vi "EventsRobotsStuck.vi"(6 "IA State Input":T5, 9 "Time":enum16{"Azul", "Amarelo"}(ring), 10 "Single frame":T1 {"robots_blue"."height" format="%+4.3f"; "robots_blue"."pixel_y" format="%+4.3f"; "robots_blue"."pixel_x" format="%+4.3f"; "robots_blue"."orientation" format="%+4.3f"; "robots_blue"."y" format="%+4.3f"; "robots_blue"."confidence" format="%4.3f"; "robots_blue"."x" format="%+4.3f"; "robots_yellow"."height" format="%+4.3f"; "robots_yellow"."pixel_y" format="%+4.3f"; "robots_yellow"."pixel_x" format="%+4.3f"; "robots_yellow"."orientation" format="%+4.3f"; "robots_yellow"."y" format="%+4.3f"; "robots_yellow"."confidence" format="%4.3f"; "robots_yellow"."x" format="%+4.3f"}, 11 "fps":dbl) -> ()   [LabVIEW 2017]
uses:
  Core/AI Input.ctl
  Core/AI Robot.ctl
  Intel/Functions Enum.ctl
  Intel/AttackerStates.ctl
  Path Planning/RRT/PathDests.ctl
  Path Planning/RRT/PathDest.ctl
  Core/AI Ball.ctl
  Core/Field Size.ctl
  Core/AI Judge.ctl
  Intel/Command Enum.ctl
  Events.ctl
  SSL Detection Frame.ctl
  SSL Detection Robot.ctl
  <vilib>/Analysis/Matrix/Datatypes/RealMatrix.ctl
  SSL Detection Ball.ctl
  <vilib>/Analysis/Matrix/NI_Matrix.lvlib
panel:
  out "Robots Stucked":cluster{"ID":i32, "Relative error":dbl}[](array[cluster])
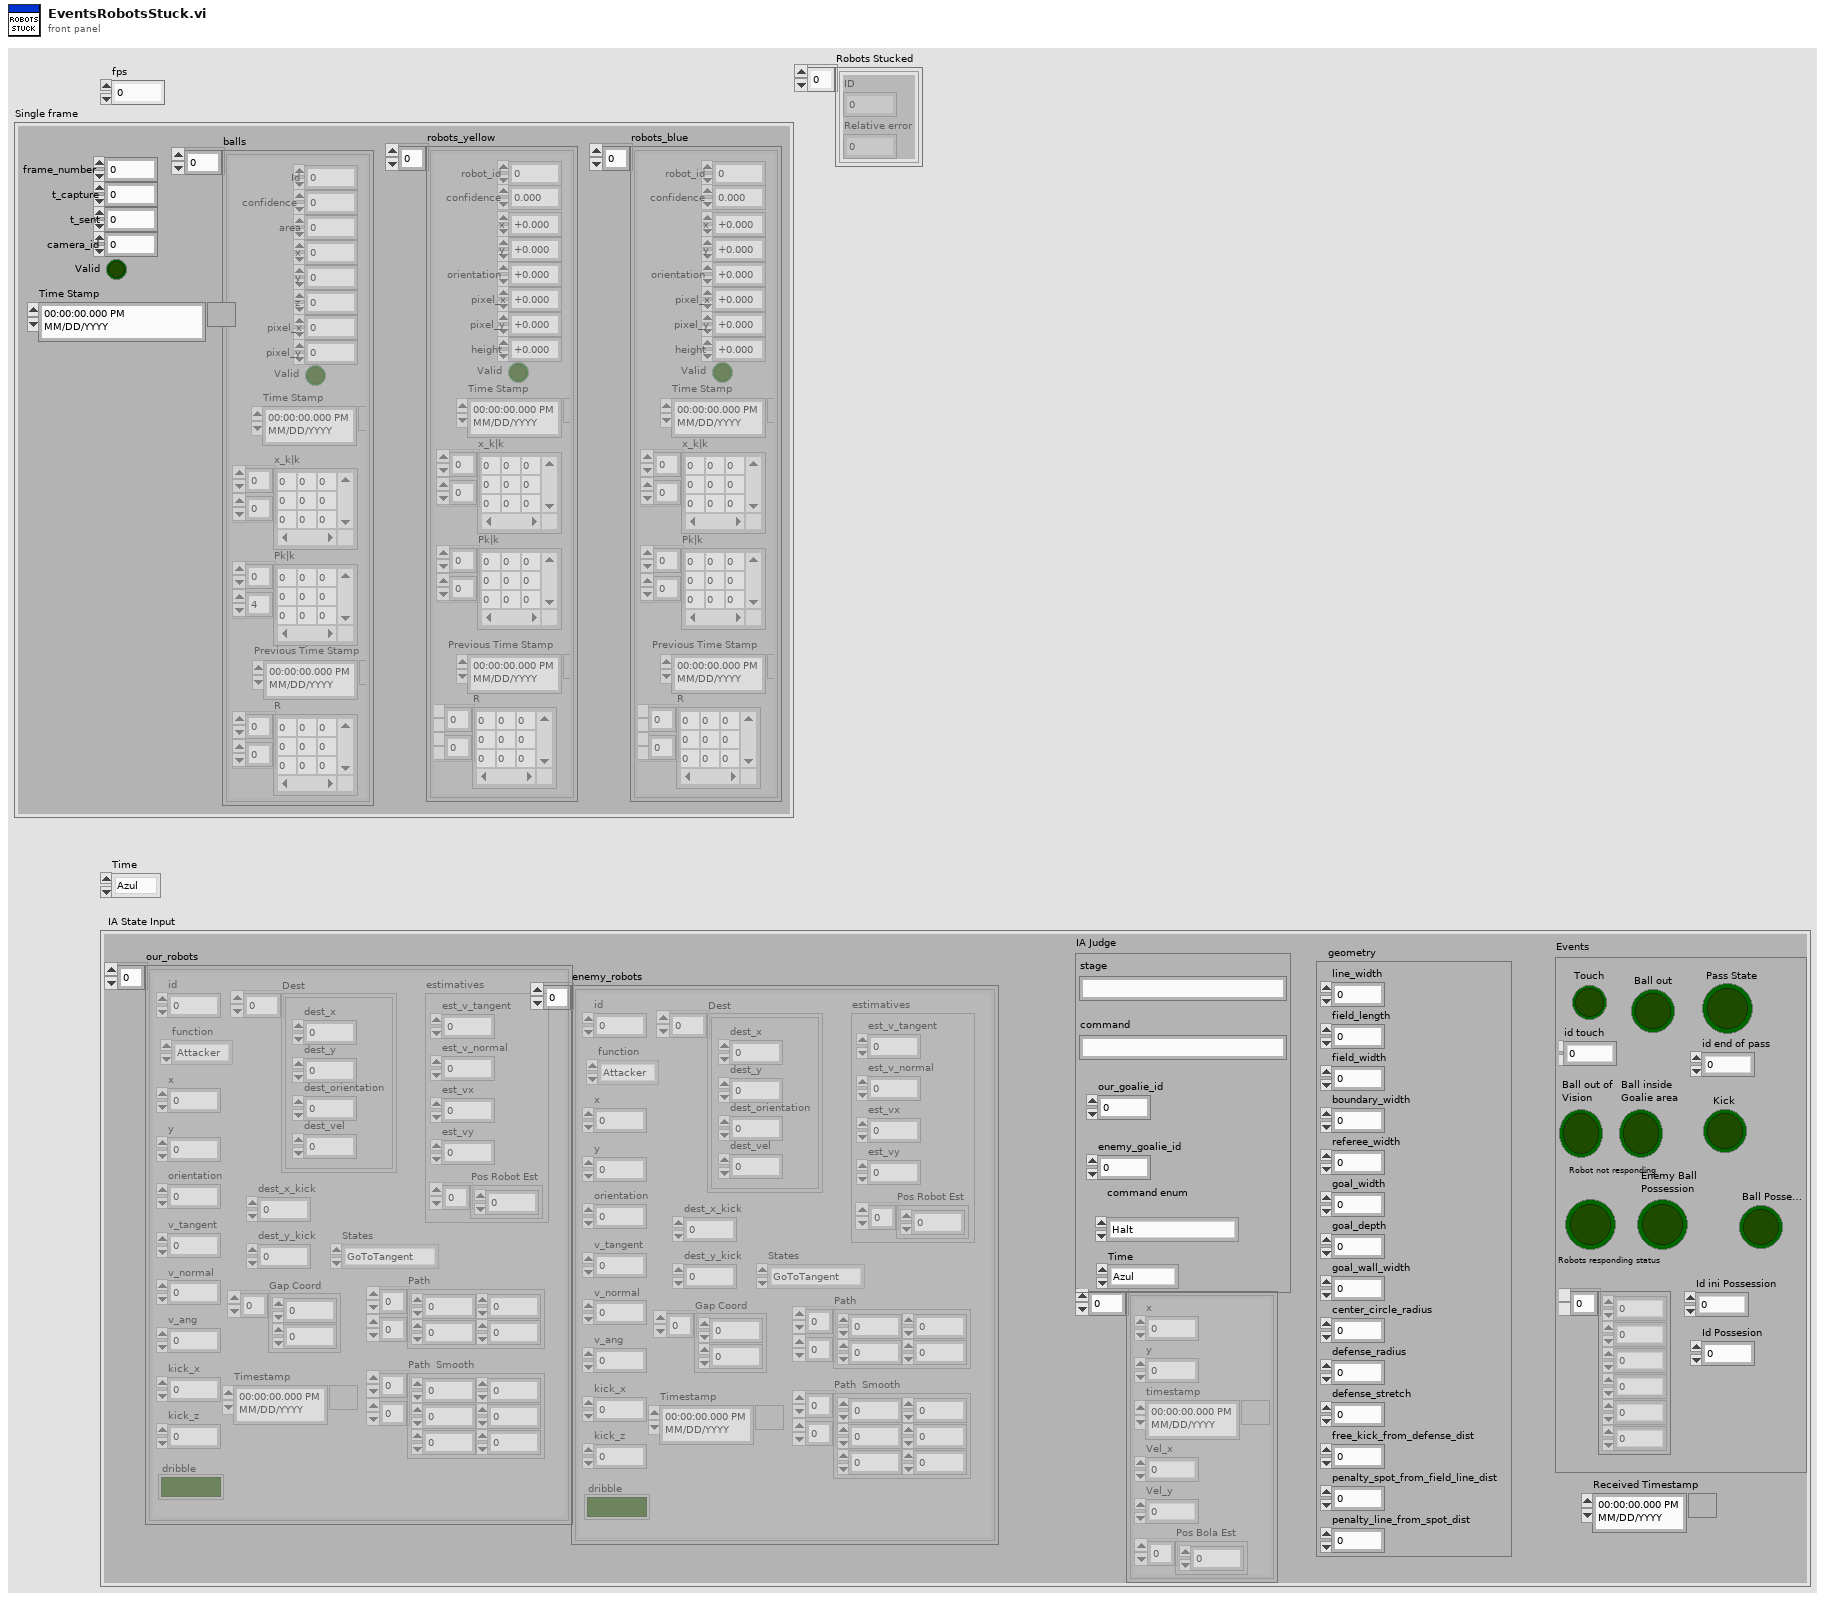
[diagram p1: front panel]
types:
  T1 = typedef "SSL Detection Frame.ctl" = cluster{"frame_number":u32, "t_capture":dbl, "t_sent":dbl, "camera_id":u32, "robots_yellow":T2[], "robots_blue":T2[], "balls":T4[], "Valid":bool, "Time Stamp":timestamp}
  T2 = typedef "SSL Detection Robot.ctl" = cluster{"x":sgl, "robot_id":u32, "confidence":sgl, "y":sgl, "orientation":sgl, "pixel_x":sgl, "pixel_y":sgl, "height":sgl, "Valid":bool, "Time Stamp":timestamp, "x_k|k":T3, "Pk|k":T3, "Previous Time Stamp":timestamp, "R":T3}
  T3 = typedef "NI_Matrix.lvlib/RealMatrix.ctl" = dbl[][]
  T4 = typedef "SSL Detection Ball.ctl" = cluster{"x":sgl, "area":u32, "confidence":sgl, "y":sgl, "z":sgl, "pixel_x":sgl, "pixel_y":sgl, "Valid":bool, "Time Stamp":timestamp, "x_k|k":T3, "Pk|k":T3, "Id":u32, "Previous Time Stamp":timestamp, "R":T3}
  T5 = typedef "AI Input.ctl" = cluster{"our_robots":T6[], "enemy_robots":T6[], "balls":T11[], "geometry":T12, "IA Judge":T13, "Received Timestamp":timestamp, "Events":T15}
  T6 = typedef "AI Robot.ctl" = cluster{"id":u32, "function":T7, "x":dbl, "y":dbl, "orientation":dbl, "v_tangent":dbl, "v_normal":dbl, "v_ang":dbl, "kick_x":dbl, "kick_z":dbl, "dribble":bool, "Timestamp":timestamp, "estimatives":cluster{"est_v_tangent":dbl, "est_v_normal":dbl, "est_vx":dbl, "est_vy":dbl, "Pos Robot Est":dbl[]}, "dest_x_kick":dbl, "dest_y_kick":dbl, "Gap Coord":dbl[], "States":T8, "Path ":dbl[][], "Path  Smooth":dbl[][], "Dest":T9}
  T7 = typedef "Functions Enum.ctl" = enum16{"Attacker", "Goalie", "Defender", "Striker", "Goto 0", "Dummy", "Kicker", "ZigZag"}
  T8 = typedef "AttackerStates.ctl" = enum16{"Pass", "GoToTangent", "BallGetting", "GoToKick", ""}
  T9 = typedef "PathDests.ctl" = T10[]
  T10 = typedef "PathDest.ctl" = cluster{"dest_x":dbl, "dest_y":dbl, "dest_orientation":dbl, "dest_vel":dbl}
  T11 = typedef "AI Ball.ctl" = cluster{"x":dbl, "y":dbl, "timestamp":timestamp, "Vel_x":dbl, "Vel_y":dbl, "Pos Bola Est":dbl[]}
  T12 = typedef "Field Size.ctl" = cluster{"line_width":u32, "field_length":u32, "field_width":u32, "boundary_width":u32, "referee_width":u32, "goal_width":u32, "goal_depth":u32, "goal_wall_width":u32, "center_circle_radius":u32, "defense_radius":u32, "defense_stretch":u32, "free_kick_from_defense_dist":u32, "penalty_spot_from_field_line_dist":u32, "penalty_line_from_spot_dist":u32}
  T13 = typedef "AI Judge.ctl" = cluster{"stage":string, "command":string, "our_goalie_id":dbl, "enemy_goalie_id":dbl, "command enum":T14, "Time":enum16{"Azul", "Amarelo"}}
  T14 = typedef "Command Enum.ctl" = enum16{"Halt", "Stop", "Force Start", "PKA Normal Start", "Prepare Kickoff Ally", "PKE Normal Start", "Prepare Kickoff Enemy", "Prepare Penalty Ally", "PPA Normal Start", "Prepare Penalty Enemy", "PPE Normal Start", "Direct Free Enemy", "Direct Free Ally", "Indirect Free Enemy", "Indirect Free Ally", "Timeout Enemy", "Timeout Ally", "Goal Enemy", "Goal Ally", "Ball Placement Enemy", "Ball Placement Ally", "Normal Half Time", "Extra Time Break", "Extra Half Time", "None", "Post Game"}
  T15 = typedef "Events.ctl" = cluster{"Touch":bool, "Ball out":bool, "id touch":dbl, "Ball out of \nVision":bool, "Ball inside \nGoalie area":bool, "Robot not responding":bool, "Robots responding status":dbl[], "Enemy Ball \nPossession":bool, "Pass State":bool, "id end of pass":dbl, "Kick":bool, "Id ini Possession":dbl, "Ball Possesion":bool, "Id Possesion":dbl}
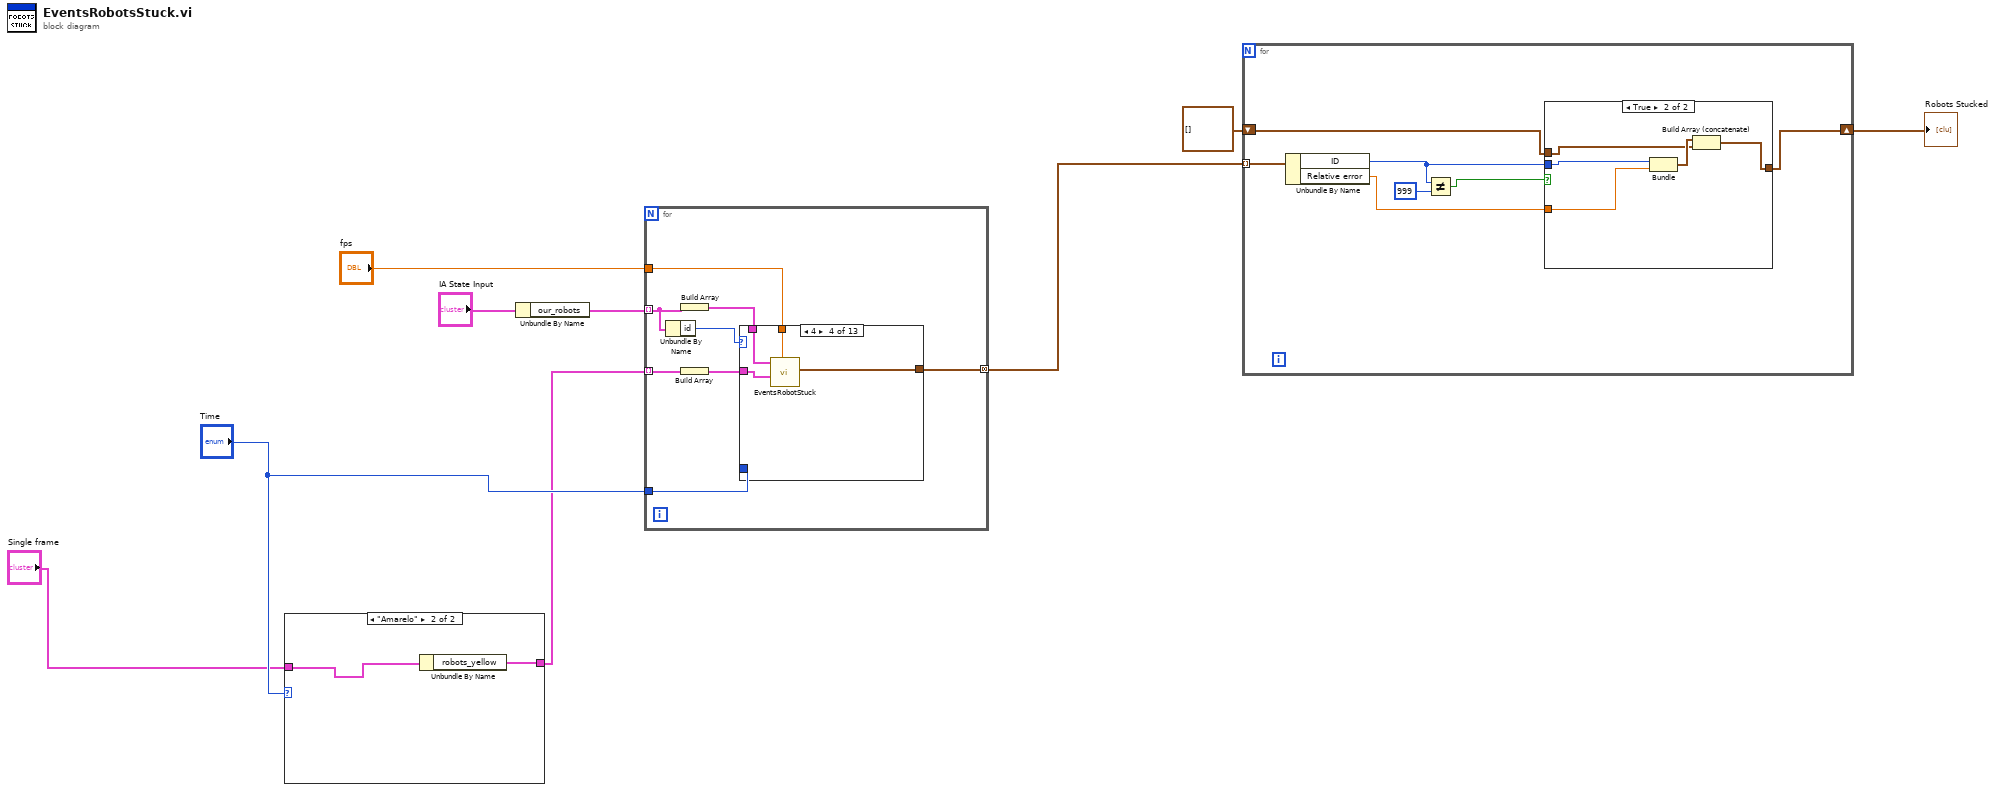
[diagram p0: block diagram]
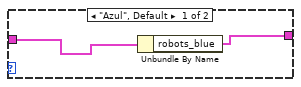
[diagram p3: hidden frame]
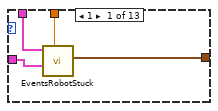
[diagram p4: hidden frame]
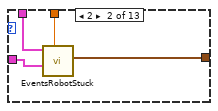
[diagram p5: hidden frame]
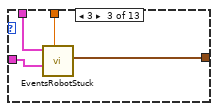
[diagram p6: hidden frame]
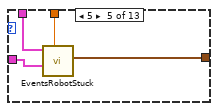
[diagram p7: hidden frame]
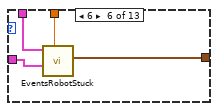
[diagram p8: hidden frame]
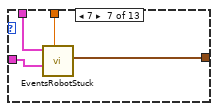
[diagram p9: hidden frame]
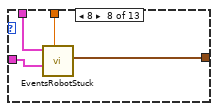
[diagram p10: hidden frame]
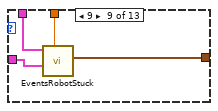
[diagram p11: hidden frame]
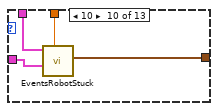
[diagram p12: hidden frame]
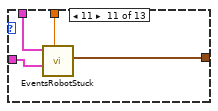
[diagram p13: hidden frame]
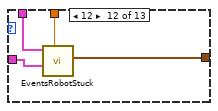
[diagram p14: hidden frame]
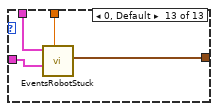
[diagram p15: hidden frame]
diagram:
  n1 = case shown="\"Amarelo\"" "Time" {
    tunnel: "Single frame" -> [w10 w12]
    tunnel: [w11 w13] -> w5
    frame "Azul", Default {
      n2 = Unbundle By Name(w10) -> ("robots_blue"=w11:T2[])
    }
    frame "Amarelo" {
      n3 = Unbundle By Name(w12) -> ("robots_yellow"=w13:T2[])
    }
  }
  n4 = Unbundle By Name("IA State Input") -> ("our_robots"=w7:T6[])
  n5 = for {
    tunnel: "fps" -> [w21]
    tunnel: "Time" -> [w20]
    tunnel: w7 -> [w17] mode=indexing
    tunnel: w5 -> [w15] mode=indexing
    tunnel: [w14] -> w3 mode=concatenating
    n6 = Unbundle By Name(w17) -> ("id"=w16:u32)
    n7 = Build Array(w17) -> (w18:T6[])
    n8 = Build Array(w15) -> (w19:T2[])
    n9 = case shown="4" w16 {
      tunnel: w21 -> [w25 w29 w33 w37 w41 w45 w49 w53 w57 w61 w65 w69 w73]
      tunnel: w20 -> [_ _ _ _ _ _ _ _ _ _ _ _ _]
      tunnel: w19 -> [w23 w27 w31 w35 w39 w43 w47 w51 w55 w59 w63 w67 w71]
      tunnel: w18 -> [w24 w28 w32 w36 w40 w44 w48 w52 w56 w60 w64 w68 w72]
      tunnel: [w22 w26 w30 w34 w38 w42 w46 w50 w54 w58 w62 w66 w70] -> w14
      frame 1 {
        n10 = call "EventsRobotStuck.vi"("our_robots"=w24, "Our_Robots frame"=w23, "FPS"=w25) -> ("Array"=w22:cluster{"ID":i32, "Relative error":dbl}[])  [unwired: 7 in]
      }
      frame 2 {
        n11 = call "EventsRobotStuck.vi"("our_robots"=w28, "Our_Robots frame"=w27, "FPS"=w29) -> ("Array"=w26:cluster{"ID":i32, "Relative error":dbl}[])  [unwired: 7 in]
      }
      frame 3 {
        n12 = call "EventsRobotStuck.vi"("our_robots"=w32, "Our_Robots frame"=w31, "FPS"=w33) -> ("Array"=w30:cluster{"ID":i32, "Relative error":dbl}[])  [unwired: 7 in]
      }
      frame 4 {
        n13 = call "EventsRobotStuck.vi"("our_robots"=w36, "Our_Robots frame"=w35, "FPS"=w37) -> ("Array"=w34:cluster{"ID":i32, "Relative error":dbl}[])  [unwired: 7 in]
      }
      frame 5 {
        n14 = call "EventsRobotStuck.vi"("our_robots"=w40, "Our_Robots frame"=w39, "FPS"=w41) -> ("Array"=w38:cluster{"ID":i32, "Relative error":dbl}[])  [unwired: 7 in]
      }
      frame 6 {
        n15 = call "EventsRobotStuck.vi"("our_robots"=w44, "Our_Robots frame"=w43, "FPS"=w45) -> ("Array"=w42:cluster{"ID":i32, "Relative error":dbl}[])  [unwired: 7 in]
      }
      frame 7 {
        n16 = call "EventsRobotStuck.vi"("our_robots"=w48, "Our_Robots frame"=w47, "FPS"=w49) -> ("Array"=w46:cluster{"ID":i32, "Relative error":dbl}[])  [unwired: 7 in]
      }
      frame 8 {
        n17 = call "EventsRobotStuck.vi"("our_robots"=w52, "Our_Robots frame"=w51, "FPS"=w53) -> ("Array"=w50:cluster{"ID":i32, "Relative error":dbl}[])  [unwired: 7 in]
      }
      frame 9 {
        n18 = call "EventsRobotStuck.vi"("our_robots"=w56, "Our_Robots frame"=w55, "FPS"=w57) -> ("Array"=w54:cluster{"ID":i32, "Relative error":dbl}[])  [unwired: 7 in]
      }
      frame 10 {
        n19 = call "EventsRobotStuck.vi"("our_robots"=w60, "Our_Robots frame"=w59, "FPS"=w61) -> ("Array"=w58:cluster{"ID":i32, "Relative error":dbl}[])  [unwired: 7 in]
      }
      frame 11 {
        n20 = call "EventsRobotStuck.vi"("our_robots"=w64, "Our_Robots frame"=w63, "FPS"=w65) -> ("Array"=w62:cluster{"ID":i32, "Relative error":dbl}[])  [unwired: 7 in]
      }
      frame 12 {
        n21 = call "EventsRobotStuck.vi"("our_robots"=w68, "Our_Robots frame"=w67, "FPS"=w69) -> ("Array"=w66:cluster{"ID":i32, "Relative error":dbl}[])  [unwired: 7 in]
      }
      frame 0, Default {
        n22 = call "EventsRobotStuck.vi"("our_robots"=w72, "Our_Robots frame"=w71, "FPS"=w73) -> ("Array"=w70:cluster{"ID":i32, "Relative error":dbl}[])  [unwired: 7 in]
      }
    }
  }
  n23 = for {
    tunnel: w3 -> [w80] mode=indexing
    shift-right: [w76] -> w1
    shift-left: cluster{"ID":i32, "Relative error":dbl}[] [] -> [w75]
    n24 = Unbundle By Name(w80) -> ("ID"=w77:i32, "Relative error"=w74:dbl)
    n25 = Not Equal?(x=w77, y=u32 999) -> (x != y?=w78:bool)
    n26 = case shown="True" w78 {
      tunnel: [w81 w84] -> w76
      tunnel: w77 -> [_ w86]
      tunnel: w75 -> [w81 w82]
      tunnel: w74 -> [_ w85]
      frame False {
      }
      frame True {
        n27 = Bundle("ID"=w86, "Relative error"=w85) -> (w83:cluster{"ID":i32, "Relative error":dbl})  [unwired: 1 in]
        n28 = Build Array (concatenate)(w83, w82) -> (w84:cluster{"ID":i32, "Relative error":dbl}[])
      }
    }
  }
  "Robots Stucked" <- w1
